vi "JSON Type Match.vi"(8 "error in (no error)":errorcluster, 9 "JSON Type":T1, 10 "JSON Value":string, 11 "Type":variant) -> (0 "error out":errorcluster, 1 "Types Match":bool, 2 "Variant Data String":string)   [LabVIEW 2011, in "LV JSON.lvlib"]
uses:
  LV JSON.lvlib
  <vilib>/Utility/VariantDataType/VariantType.lvlib
  <vilib>/picture/picture.llb/imagedata.ctl
  controls/JSON type.ctl
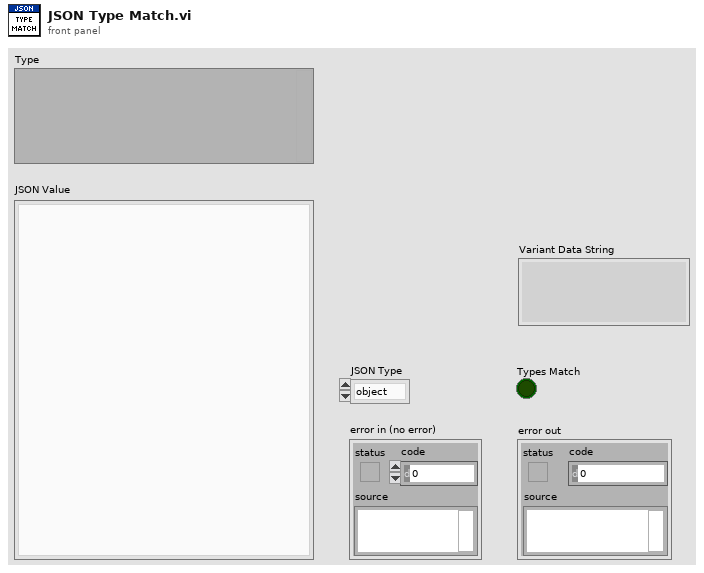
[diagram p1: front panel]
types:
  T1 = typedef "LV JSON.lvlib/JSON type.ctl" = enum16{"object", "array", "number", "string", "boolean", "null"}
  T2 = typedef "VariantType.lvlib/Type.ctl" = enum8{"Invalid Type", "Void", "I8", "I16", "I32", "I64", "U8", "U16", "U32", "U64", "Single Float", "Double Float", "Extended Float", "Single Complex", "Double Complex", "Extended Complex", "Enum U8", "Enum U16", "Enum U32", "Enum U64", "Single Float With Unit", "Double Float With Unit", "Extended Float With Unit", "Single Complex with Unit", "Double Complex with Unit", "Extended Complex with Unit", "Boolean", "String", "Path", "Picture", "Tag", "Array", "Cluster", "Variant", "LV Variant", "Waveform", "Timestamp", "Digital Waveform", "Digital Data", "ExpressData", "Refnum", "External Data", "VI", "Poly VI", "LabVIEW Class Instance", "Fixed Point"}
  T3 = typedef "imagedata.ctl" = cluster{"image type":i32, "image depth":i32, "image":u8[], "mask":u8[], "colors":u32[], "Rectangle":cluster{"left":i16, "top":i16, "right":i16, "bottom":i16}}
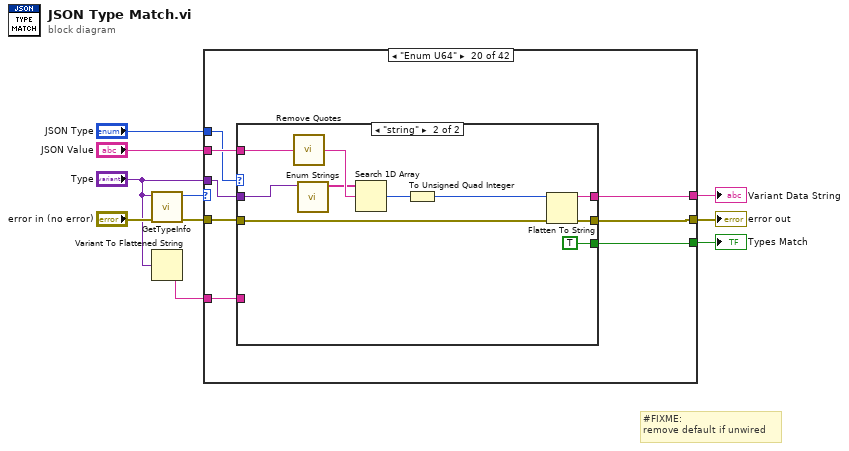
[diagram p0: block diagram]
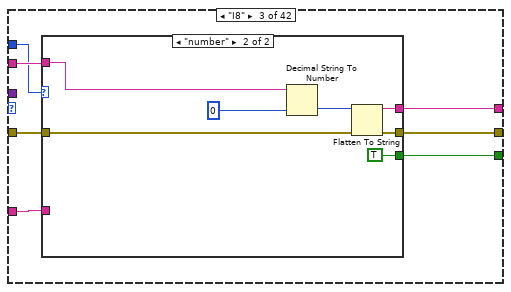
[diagram p4: hidden frame]
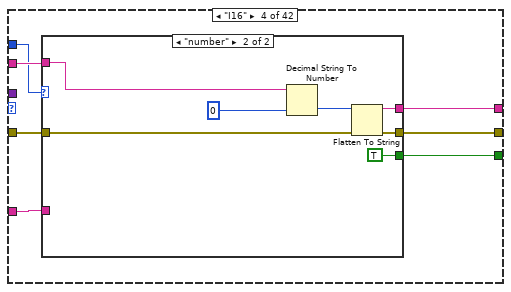
[diagram p6: hidden frame]
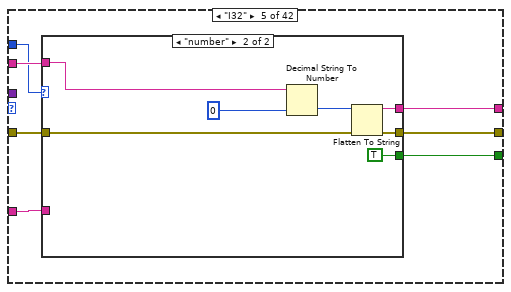
[diagram p8: hidden frame]
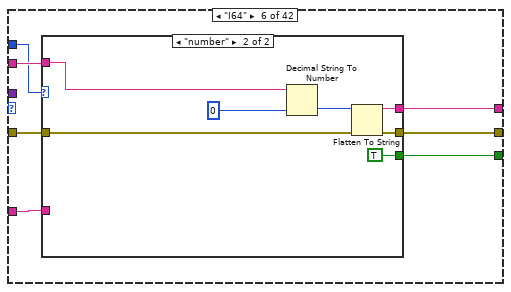
[diagram p10: hidden frame]
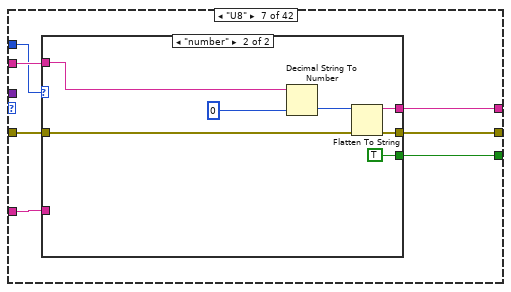
[diagram p12: hidden frame]
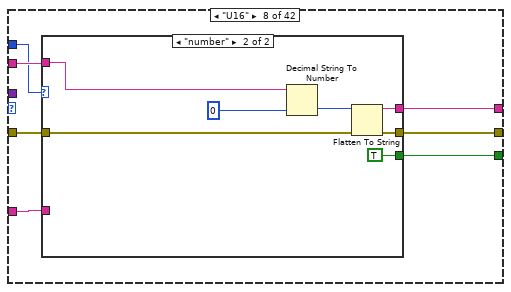
[diagram p14: hidden frame]
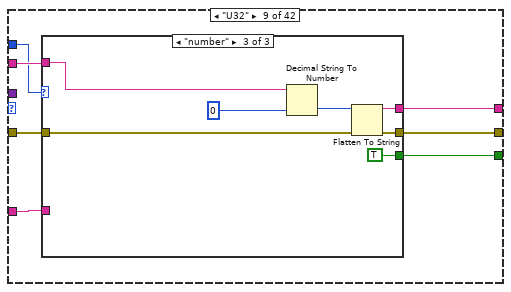
[diagram p16: hidden frame]
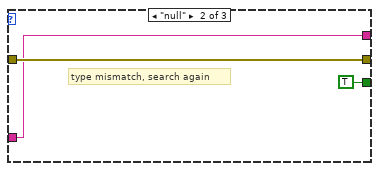
[diagram p18: hidden frame]
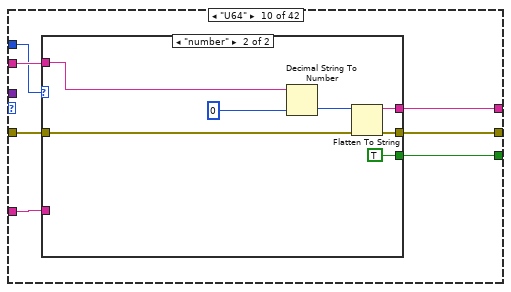
[diagram p19: hidden frame]
diagram:
  # "#FIXME:\nremove default if unwired"
  n1 = call <vilib>:"GetTypeInfo.vi"("error in (no error)"="error in (no error)", "Variant"="Type") -> ("error out"=w8:errorcluster, "Type Enum"=w7:T2)  [unwired: 5 in, 3 out]
  n2 = Variant To Flattened String(Variant="Type") -> (data string=w4:string)  [unwired: 1 out]
  n3 = case shown="\"Enum U64\"" w7 {
    tunnel: [_ _ w14 w30 w46 w62 w78 w94 w110 w129 w144 w164 w180 _ _ _ w191 w211 w231 w251 _ _ w272 w292 w296 w312 _ w326 w489 _ _ _ w510 _ _ _ w529 _ _ _ _ _] -> w1
    tunnel: w8 -> [_ _ w17 w33 w49 w65 w81 w97 w113 w132 w146 w163 w179 _ _ _ w196 w216 w236 w256 _ _ w274 w293 w298 w319 _ w328 w488 _ _ _ w509 _ _ _ w531 _ _ _ _ _]
    tunnel: [_ _ w13 w29 w45 w61 w77 w93 w109 w128 w142 w162 w178 _ _ _ w192 w212 w232 w252 _ _ w271 w291 w295 w313 _ w327 w487 _ _ _ w508 _ _ _ w531 _ _ _ _ _] -> w2
    tunnel: "Type" -> [_ _ _ _ _ _ _ _ _ _ _ _ _ _ _ _ w190 w210 w230 w250 _ _ _ _ _ _ _ w325 w482 _ _ _ _ _ _ _ _ _ _ _ _ _]
    tunnel: "JSON Value" -> [_ _ w16 w32 w48 w64 w80 w96 w112 w131 w148 w160 w176 _ _ _ w197 w217 w237 w257 _ _ w276 w289 w300 w320 _ w324 w485 _ _ _ w512 _ _ _ _ _ _ _ _ _]
    tunnel: "JSON Type" -> [_ _ w15 w31 w47 w63 w79 w95 w111 w130 w147 w161 w177 _ _ _ w194 w214 w234 w254 _ _ w275 _ w299 _ _ w323 w486 _ _ _ w511 _ _ _ _ _ _ _ _ _]
    tunnel: w4 -> [_ _ w11 w27 w43 w59 w75 w91 w107 w126 w145 w159 w175 _ _ _ w195 w215 w235 w255 _ _ w273 _ w297 _ _ w322 w484 _ _ _ w507 _ _ _ w529 _ _ _ _ _]
    tunnel: [_ _ w12 w28 w44 w60 w76 w92 w108 w127 w143 w158 w174 _ _ _ w193 w213 w233 w253 _ _ w270 TRUE w294 TRUE _ w321 w483 _ _ _ w513 _ _ _ TRUE _ _ _ _ _] -> w3
    frame "Invalid Type", Default {
    }
    frame "Void" {
    }
    frame "I8" {
      n4 = case shown="\"number\"" w15 {
        tunnel: [w18 w24] -> w14
        tunnel: w17 -> [w19 w23]
        tunnel: [w19 w22] -> w13
        tunnel: w16 -> [_ w21]
        tunnel: w11 -> [w18 _]
        tunnel: [_ TRUE] -> w12
        frame Default {
          # "type mismatch, search again"
        }
        frame "number" {
          n5 = Decimal String To Number(string=w21, default (0L)=i8 0 ("default (0 DBL)")) -> (number=w25:i8)  [unwired: 1 in, 1 out]
          n6 = Flatten To String(anything=w25, error in (no error)=w23) -> (data string=w24:string, error out=w22:errorcluster)  [unwired: 2 in, 1 out]
        }
      }
    }
    frame "I16" {
      n7 = case shown="\"number\"" w31 {
        tunnel: [w34 w40] -> w30
        tunnel: w33 -> [w35 w39]
        tunnel: [w35 w38] -> w29
        tunnel: w32 -> [_ w37]
        tunnel: w27 -> [w34 _]
        tunnel: [_ TRUE] -> w28
        frame Default {
          # "type mismatch, search again"
        }
        frame "number" {
          n8 = Decimal String To Number(string=w37, default (0L)=i16 0 ("default (0 DBL)")) -> (number=w41:i16)  [unwired: 1 in, 1 out]
          n9 = Flatten To String(anything=w41, error in (no error)=w39) -> (data string=w40:string, error out=w38:errorcluster)  [unwired: 2 in, 1 out]
        }
      }
    }
    frame "I32" {
      n10 = case shown="\"number\"" w47 {
        tunnel: [w50 w56] -> w46
        tunnel: w49 -> [w51 w55]
        tunnel: [w51 w54] -> w45
        tunnel: w48 -> [_ w53]
        tunnel: w43 -> [w50 _]
        tunnel: [_ TRUE] -> w44
        frame Default {
          # "type mismatch, search again"
        }
        frame "number" {
          n11 = Decimal String To Number(string=w53, default (0L)=0 ("default (0 DBL)")) -> (number=w57:i32)  [unwired: 1 in, 1 out]
          n12 = Flatten To String(anything=w57, error in (no error)=w55) -> (data string=w56:string, error out=w54:errorcluster)  [unwired: 2 in, 1 out]
        }
      }
    }
    frame "I64" {
      n13 = case shown="\"number\"" w63 {
        tunnel: [w66 w72] -> w62
        tunnel: w65 -> [w67 w71]
        tunnel: [w67 w70] -> w61
        tunnel: w64 -> [_ w69]
        tunnel: w59 -> [w66 _]
        tunnel: [_ TRUE] -> w60
        frame Default {
          # "type mismatch, search again"
        }
        frame "number" {
          n14 = Decimal String To Number(string=w69, default (0L)=i64 0 ("default (0 DBL)")) -> (number=w73:i64)  [unwired: 1 in, 1 out]
          n15 = Flatten To String(anything=w73, error in (no error)=w71) -> (data string=w72:string, error out=w70:errorcluster)  [unwired: 2 in, 1 out]
        }
      }
    }
    frame "U8" {
      n16 = case shown="\"number\"" w79 {
        tunnel: [w82 w88] -> w78
        tunnel: w81 -> [w83 w87]
        tunnel: [w83 w86] -> w77
        tunnel: w80 -> [_ w85]
        tunnel: w75 -> [w82 _]
        tunnel: [_ TRUE] -> w76
        frame Default {
          # "type mismatch, search again"
        }
        frame "number" {
          n17 = Decimal String To Number(string=w85, default (0L)=u8 0 ("default (0 DBL)")) -> (number=w89:u8)  [unwired: 1 in, 1 out]
          n18 = Flatten To String(anything=w89, error in (no error)=w87) -> (data string=w88:string, error out=w86:errorcluster)  [unwired: 2 in, 1 out]
        }
      }
    }
    frame "U16" {
      n19 = case shown="\"number\"" w95 {
        tunnel: [w98 w104] -> w94
        tunnel: w97 -> [w99 w103]
        tunnel: [w99 w102] -> w93
        tunnel: w96 -> [_ w101]
        tunnel: w91 -> [w98 _]
        tunnel: [_ TRUE] -> w92
        frame Default {
          # "type mismatch, search again"
        }
        frame "number" {
          n20 = Decimal String To Number(string=w101, default (0L)=u16 0 ("default (0 DBL)")) -> (number=w105:u16)  [unwired: 1 in, 1 out]
          n21 = Flatten To String(anything=w105, error in (no error)=w103) -> (data string=w104:string, error out=w102:errorcluster)  [unwired: 2 in, 1 out]
        }
      }
    }
    frame "U32" {
      n22 = case shown="\"number\"" w111 {
        tunnel: [w114 w117 w123] -> w110
        tunnel: w113 -> [w115 w118 w122]
        tunnel: [w115 w118 w121] -> w109
        tunnel: w112 -> [_ _ w120]
        tunnel: w107 -> [w114 w117 _]
        tunnel: [_ TRUE TRUE] -> w108
        frame Default {
          # "type mismatch, search again"
        }
        frame "null" {
          # "type mismatch, search again"
        }
        frame "number" {
          n23 = Decimal String To Number(string=w120, default (0L)=u32 0 ("default (0 DBL)")) -> (number=w124:u32)  [unwired: 1 in, 1 out]
          n24 = Flatten To String(anything=w124, error in (no error)=w122) -> (data string=w123:string, error out=w121:errorcluster)  [unwired: 2 in, 1 out]
        }
      }
    }
    frame "U64" {
      n25 = case shown="\"number\"" w130 {
        tunnel: [w133 w139] -> w129
        tunnel: w132 -> [w134 w138]
        tunnel: [w134 w137] -> w128
        tunnel: w131 -> [_ w136]
        tunnel: w126 -> [w133 _]
        tunnel: [_ TRUE] -> w127
        frame Default {
          # "type mismatch, search again"
        }
        frame "number" {
          n26 = Decimal String To Number(string=w136, default (0L)=u64 0 ("default (0 DBL)")) -> (number=w140:u64)  [unwired: 1 in, 1 out]
          n27 = Flatten To String(anything=w140, error in (no error)=w138) -> (data string=w139:string, error out=w137:errorcluster)  [unwired: 2 in, 1 out]
        }
      }
    }
    frame "Single Float", "Single Float With Unit" {
      n28 = case shown="\"number\"" w147 {
        tunnel: [w149 w155] -> w144
        tunnel: w146 -> [w150 w154]
        tunnel: [w150 w153] -> w142
        tunnel: w148 -> [_ w152]
        tunnel: w145 -> [w149 _]
        tunnel: [_ TRUE] -> w143
        frame Default {
          # "type mismatch, search again"
        }
        frame "number" {
          n29 = Fract/Exp String To Number(string=w152, default (0 dbl)=sgl 0.0 ("default (0 DBL)")) -> (number=w156:sgl)  [unwired: 2 in, 1 out]
          n30 = Flatten To String(anything=w156, error in (no error)=w154) -> (data string=w155:string, error out=w153:errorcluster)  [unwired: 2 in, 1 out]
        }
      }
    }
    frame "Double Float", "Double Float With Unit" {
      n31 = case shown="\"number\"" w161 {
        tunnel: [w165 w171] -> w164
        tunnel: w163 -> [w166 w170]
        tunnel: [w166 w169] -> w162
        tunnel: w160 -> [_ w168]
        tunnel: w159 -> [w165 _]
        tunnel: [_ TRUE] -> w158
        frame Default {
          # "type mismatch, search again"
        }
        frame "number" {
          n32 = Fract/Exp String To Number(string=w168, default (0 dbl)=0.0 ("default (0 DBL)")) -> (number=w172:dbl)  [unwired: 2 in, 1 out]
          n33 = Flatten To String(anything=w172, error in (no error)=w170) -> (data string=w171:string, error out=w169:errorcluster)  [unwired: 2 in, 1 out]
        }
      }
    }
    frame "Extended Float", "Extended Float With Unit" {
      n34 = case shown="\"number\"" w177 {
        tunnel: [w181 w187] -> w180
        tunnel: w179 -> [w182 w186]
        tunnel: [w182 w185] -> w178
        tunnel: w176 -> [_ w184]
        tunnel: w175 -> [w181 _]
        tunnel: [_ TRUE] -> w174
        frame Default {
          # "type mismatch, search again"
        }
        frame "number" {
          n35 = Fract/Exp String To Number(string=w184, default (0 dbl)=ext 0.0 ("default (0 DBL)")) -> (number=w188:ext)  [unwired: 2 in, 1 out]
          n36 = Flatten To String(anything=w188, error in (no error)=w186) -> (data string=w187:string, error out=w185:errorcluster)  [unwired: 2 in, 1 out]
        }
      }
    }
    frame "Single Complex" {
    }
    frame "Double Complex" {
    }
    frame "Extended Complex" {
    }
    frame "Enum U8" {
      n37 = case shown="\"string\"" w194 {
        tunnel: [w198 w207] -> w191
        tunnel: w196 -> [w199 w200]
        tunnel: [w199 w208] -> w192
        tunnel: w197 -> [_ w204]
        tunnel: w195 -> [w198 _]
        tunnel: [_ TRUE] -> w193
        tunnel: w190 -> [_ w202]
        frame Default {
          # "type mismatch, search again"
        }
        frame "string" {
          n38 = call "Remove Quotes.vi"("String"=w204) -> ("String without Quotes"=w203:string)
          n39 = call "Enum Strings.vi"("Enum"=w202) -> ("Strings"=w201:string[])  [unwired: 8 in, 2 out]
          n40 = Search 1D Array(1D array=w201, element=w203) -> (index of element=w206:i32)  [unwired: 1 in]
          n41 = To Unsigned Byte Integer(number=w206) -> (unsigned 8bit integer=w205:u8)
          n42 = Flatten To String(anything=w205, error in (no error)=w200) -> (data string=w207:string, error out=w208:errorcluster)  [unwired: 2 in, 1 out]
        }
      }
    }
    frame "Enum U16" {
      n43 = case shown="\"string\"" w214 {
        tunnel: [w218 w227] -> w211
        tunnel: w216 -> [w219 w220]
        tunnel: [w219 w228] -> w212
        tunnel: w217 -> [_ w224]
        tunnel: w215 -> [w218 _]
        tunnel: [_ TRUE] -> w213
        tunnel: w210 -> [_ w222]
        frame Default {
          # "type mismatch, search again"
        }
        frame "string" {
          n44 = call "Remove Quotes.vi"("String"=w224) -> ("String without Quotes"=w223:string)
          n45 = call "Enum Strings.vi"("Enum"=w222) -> ("Strings"=w221:string[])  [unwired: 8 in, 2 out]
          n46 = Search 1D Array(1D array=w221, element=w223) -> (index of element=w226:i32)  [unwired: 1 in]
          n47 = To Unsigned Word Integer(number=w226) -> (unsigned 16bit integer=w225:u16)
          n48 = Flatten To String(anything=w225, error in (no error)=w220) -> (data string=w227:string, error out=w228:errorcluster)  [unwired: 2 in, 1 out]
        }
      }
    }
    frame "Enum U32" {
      n49 = case shown="\"string\"" w234 {
        tunnel: [w238 w247] -> w231
        tunnel: w236 -> [w239 w240]
        tunnel: [w239 w248] -> w232
        tunnel: w237 -> [_ w244]
        tunnel: w235 -> [w238 _]
        tunnel: [_ TRUE] -> w233
        tunnel: w230 -> [_ w241]
        frame Default {
          # "type mismatch, search again"
        }
        frame "string" {
          n50 = call "Remove Quotes.vi"("String"=w244) -> ("String without Quotes"=w243:string)
          n51 = call "Enum Strings.vi"("Enum"=w241) -> ("Strings"=w242:string[])  [unwired: 8 in, 2 out]
          n52 = Search 1D Array(1D array=w242, element=w243) -> (index of element=w246:i32)  [unwired: 1 in]
          n53 = To Unsigned Long Integer(number=w246) -> (unsigned 32bit integer=w245:u32)
          n54 = Flatten To String(anything=w245, error in (no error)=w240) -> (data string=w247:string, error out=w248:errorcluster)  [unwired: 2 in, 1 out]
        }
      }
    }
    frame "Enum U64" {
      n55 = case shown="\"string\"" w254 {
        tunnel: [w258 w267] -> w251
        tunnel: w256 -> [w259 w261]
        tunnel: [w259 w268] -> w252
        tunnel: w257 -> [_ w264]
        tunnel: w255 -> [w258 _]
        tunnel: [_ TRUE] -> w253
        tunnel: w250 -> [_ w260]
        frame Default {
          # "type mismatch, search again"
        }
        frame "string" {
          n56 = call "Remove Quotes.vi"("String"=w264) -> ("String without Quotes"=w263:string)
          n57 = call "Enum Strings.vi"("Enum"=w260) -> ("Strings"=w262:string[])  [unwired: 8 in, 2 out]
          n58 = Search 1D Array(1D array=w262, element=w263) -> (index of element=w266:i32)  [unwired: 1 in]
          n59 = To Unsigned Quad Integer(1:w266) -> (0:w265:u64)
          n60 = Flatten To String(anything=w265, error in (no error)=w261) -> (data string=w267:string, error out=w268:errorcluster)  [unwired: 2 in, 1 out]
        }
      }
    }
    frame "Single Complex with Unit" {
    }
    frame "Extended Complex with Unit" {
    }
    frame "Boolean" {
      n61 = case shown="\"boolean\"" w275 {
        tunnel: [w277 w282] -> w272
        tunnel: w274 -> [w278 w280]
        tunnel: [w278 w283] -> w271
        tunnel: w276 -> [_ w285]
        tunnel: w273 -> [w277 _]
        tunnel: [_ TRUE] -> w270
        frame Default {
          # "type mismatch, search again"
        }
        frame "boolean" {
          n62 = To Lower Case(string=w285) -> (all lower case string=w279:string)
          n63 = Equal?(x=w279, y="true") -> (x = y?=w281:bool)
          n64 = Flatten To String(anything=w281, error in (no error)=w280) -> (data string=w282:string, error out=w283:errorcluster)  [unwired: 2 in, 1 out]
        }
      }
    }
    frame "String" {
      n65 = call "Remove Quotes.vi"("String"=w289) -> ("String without Quotes"=w288:string)
      n66 = call "JSON Unescape.vi"("Escaped JSON String"=w288) -> ("JSON String"=w287:string)
      n67 = Flatten To String(anything=w287, error in (no error)=w293) -> (data string=w292:string, error out=w291:errorcluster)  [unwired: 2 in, 1 out]
    }
    frame "Path" {
      n68 = case shown="\"string\"" w299 {
        tunnel: [w301 w310] -> w296
        tunnel: w298 -> [w302 w309]
        tunnel: [w302 w308] -> w295
        tunnel: w300 -> [_ w305]
        tunnel: w297 -> [w301 _]
        tunnel: [_ TRUE] -> w294
        frame Default {
          # "type mismatch, search again"
        }
        frame "string" {
          n69 = call "Remove Quotes.vi"("String"=w305) -> ("String without Quotes"=w304:string)
          n70 = call "JSON Unescape.vi"("Escaped JSON String"=w304) -> ("JSON String"=w303:string)
          n71 = String To Path(string=w303) -> (path=w306:path)
          n72 = Flatten To String(anything=w306, error in (no error)=w309) -> (data string=w310:string, error out=w308:errorcluster)  [unwired: 2 in, 1 out]
        }
      }
    }
    frame "Picture" {
      w317 = T3 {"image type"=0, "image depth"=0, "image"=[], "mask"=[], "colors"=[], "Rectangle"={"left"=0, "top"=0, "right"=0, "bottom"=0}} ("image data")
      n73 = call "JSON to Anything.vi"("error in (no error)"=w319, "JSON Object"=w320, "Type"=w317) -> ("error out"=w316:errorcluster, "Variant"=w318:variant)  [unwired: 5 in, 2 out]
      n74 = Variant To Data(error in=w316, type=w317, Variant=w318) -> (data=w314:T3, error out=w315:errorcluster)
      n75 = Flatten To String(anything=w314, error in (no error)=w315) -> (data string=w312:string, error out=w313:errorcluster)  [unwired: 2 in, 1 out]
    }
    frame "Tag" {
    }
    frame "Array" {
      n76 = case shown="\"array\"" w323 {
        tunnel: w328 -> [w330 w339]
        tunnel: [w330 w334] -> w327
        tunnel: [w329 w333] -> w326
        tunnel: w325 -> [_ w337]
        tunnel: w324 -> [_ w331]
        tunnel: w322 -> [w329 _]
        tunnel: [_ TRUE] -> w321
        frame Default {
        }
        frame "array" {
          n77 = call "JSON Parse Array.vi"("error in (no error)"=w339, "JSON Array Value"=w331, "Type"=w337) -> ("error out"=w338:errorcluster, "variant"=w335:variant, "Type Enum"=w332:T2)  [unwired: 5 in, 1 out]
          n78 = case shown="\"Cluster\"" w332 {
            tunnel: w338 -> [w340 w347 w354 w361 w368 w375 w382 w389 w396 w403 w410 w417 w424 w431 w438 w445 w452 w459 w464]
            tunnel: w335 -> [_ w346 w353 w360 w367 w374 w381 w388 w395 w402 w409 w416 w423 w430 w437 w444 w451 w458 w463]
            tunnel: [w340 w343 w350 w357 w364 w371 w378 w385 w392 w399 w406 w413 w420 w427 w434 w442 w449 w456 w460] -> w334
            tunnel: [_ w342 w349 w356 w363 w370 w377 w384 w391 w398 w405 w412 w419 w426 w433 w441 w448 w455 w461] -> w333
            tunnel: w331 -> [_ _ _ _ _ _ _ _ _ _ _ _ _ _ _ _ _ _ w462]
            frame "Invalid Type", Default {
            }
            frame "Double Float", "Double Float With Unit" {
              n79 = Variant To Data(error in=w347, type=dbl[] [], Variant=w346) -> (data=w341:dbl[], error out=w344:errorcluster)
              n80 = Flatten To String(anything=w341, error in (no error)=w344) -> (data string=w342:string, error out=w343:errorcluster)  [unwired: 2 in, 1 out]
            }
            frame "Single Float", "Single Float With Unit" {
              n81 = Variant To Data(error in=w354, type=sgl[] [], Variant=w353) -> (data=w348:sgl[], error out=w351:errorcluster)
              n82 = Flatten To String(anything=w348, error in (no error)=w351) -> (data string=w349:string, error out=w350:errorcluster)  [unwired: 2 in, 1 out]
            }
            frame "Extended Float", "Extended Float With Unit" {
              n83 = Variant To Data(error in=w361, type=ext[] [], Variant=w360) -> (data=w355:ext[], error out=w358:errorcluster)
              n84 = Flatten To String(anything=w355, error in (no error)=w358) -> (data string=w356:string, error out=w357:errorcluster)  [unwired: 2 in, 1 out]
            }
            frame "Single Complex" {
              n85 = Variant To Data(error in=w368, type=csg[] [], Variant=w367) -> (data=w362:csg[], error out=w365:errorcluster)
              n86 = Flatten To String(anything=w362, error in (no error)=w365) -> (data string=w363:string, error out=w364:errorcluster)  [unwired: 2 in, 1 out]
            }
            frame "Double Complex" {
              n87 = Variant To Data(error in=w375, type=cdb[] [], Variant=w374) -> (data=w369:cdb[], error out=w372:errorcluster)
              n88 = Flatten To String(anything=w369, error in (no error)=w372) -> (data string=w370:string, error out=w371:errorcluster)  [unwired: 2 in, 1 out]
            }
            frame "Extended Complex" {
              n89 = Variant To Data(error in=w382, type=cxt[] [], Variant=w381) -> (data=w376:cxt[], error out=w379:errorcluster)
              n90 = Flatten To String(anything=w376, error in (no error)=w379) -> (data string=w377:string, error out=w378:errorcluster)  [unwired: 2 in, 1 out]
            }
            frame "I8" {
              n91 = Variant To Data(error in=w389, type=i8[] [], Variant=w388) -> (data=w383:i8[], error out=w386:errorcluster)
              n92 = Flatten To String(anything=w383, error in (no error)=w386) -> (data string=w384:string, error out=w385:errorcluster)  [unwired: 2 in, 1 out]
            }
            frame "I16" {
              n93 = Variant To Data(error in=w396, type=i16[] [], Variant=w395) -> (data=w390:i16[], error out=w393:errorcluster)
              n94 = Flatten To String(anything=w390, error in (no error)=w393) -> (data string=w391:string, error out=w392:errorcluster)  [unwired: 2 in, 1 out]
            }
            frame "I32" {
              n95 = Variant To Data(error in=w403, type=i32[] [], Variant=w402) -> (data=w397:i32[], error out=w400:errorcluster)
              n96 = Flatten To String(anything=w397, error in (no error)=w400) -> (data string=w398:string, error out=w399:errorcluster)  [unwired: 2 in, 1 out]
            }
            frame "I64" {
              n97 = Variant To Data(error in=w410, type=i64[] [], Variant=w409) -> (data=w404:i64[], error out=w407:errorcluster)
              n98 = Flatten To String(anything=w404, error in (no error)=w407) -> (data string=w405:string, error out=w406:errorcluster)  [unwired: 2 in, 1 out]
            }
            frame "U8" {
              n99 = Variant To Data(error in=w417, type=u8[] [], Variant=w416) -> (data=w411:u8[], error out=w414:errorcluster)
              n100 = Flatten To String(anything=w411, error in (no error)=w414) -> (data string=w412:string, error out=w413:errorcluster)  [unwired: 2 in, 1 out]
            }
            frame "U16" {
              n101 = Variant To Data(error in=w424, type=u16[] [], Variant=w423) -> (data=w418:u16[], error out=w421:errorcluster)
              n102 = Flatten To String(anything=w418, error in (no error)=w421) -> (data string=w419:string, error out=w420:errorcluster)  [unwired: 2 in, 1 out]
            }
            frame "U32" {
              n103 = Variant To Data(error in=w431, type=u32[] [], Variant=w430) -> (data=w425:u32[], error out=w428:errorcluster)
              n104 = Flatten To String(anything=w425, error in (no error)=w428) -> (data string=w426:string, error out=w427:errorcluster)  [unwired: 2 in, 1 out]
            }
            frame "U64" {
              n105 = Variant To Data(error in=w438, type=u64[] [], Variant=w437) -> (data=w432:u64[], error out=w435:errorcluster)
              n106 = Flatten To String(anything=w432, error in (no error)=w435) -> (data string=w433:string, error out=w434:errorcluster)  [unwired: 2 in, 1 out]
            }
            frame "Path" {
              n107 = Variant To Data(error in=w445, type=path[] [], Variant=w444) -> (data=w440:path[], error out=w443:errorcluster)
              n108 = Flatten To String(anything=w440, error in (no error)=w443) -> (data string=w441:string, error out=w442:errorcluster)  [unwired: 2 in, 1 out]
            }
            frame "Boolean" {
              n109 = Variant To Data(error in=w452, type=bool[] [], Variant=w451) -> (data=w447:bool[], error out=w450:errorcluster)
              n110 = Flatten To String(anything=w447, error in (no error)=w450) -> (data string=w448:string, error out=w449:errorcluster)  [unwired: 2 in, 1 out]
            }
            frame "String" {
              n111 = Variant To Data(error in=w459, type=string[] [], Variant=w458) -> (data=w454:string[], error out=w457:errorcluster)
              n112 = Flatten To String(anything=w454, error in (no error)=w457) -> (data string=w455:string, error out=w456:errorcluster)  [unwired: 2 in, 1 out]
            }
            frame "Cluster" {
              n113 = disable-structure shown="Enabled" {
                disable-tunnel: w464 -> [w471 w480]
                disable-tunnel: w463 -> [w470 w481]
                disable-tunnel: w462 -> [w469 _]
                disable-tunnel: [w466 w479] -> w461
                disable-tunnel: [w465 w480] -> w460
                frame Disabled {
                  n114 = call "Cluster Elements.vi"("error in (no error)"=w471, "Cluster Variant"=w470) -> ("error out"=w472:errorcluster, "Cluster Elements"=w473:variant[])  [unwired: 8 in]
                  n115 = for {
                    tunnel: w472 -> [w478]
                    tunnel: w473 -> [w475] mode=indexing
                    tunnel: w469 -> [w474]
                    tunnel: [w477] -> w468 mode=indexing
                    tunnel: [w476] -> w467 mode=indexing
                    n116 = call "JSON to Anything.vi"("error in (no error)"=w478, "JSON Object"=w474, "Type"=w475) -> ("error out"=w477:errorcluster, "Variant Data String"=w476:string)  [unwired: 5 in, 2 out]
                  }
                  n117 = Concatenate Strings(w467) -> (w466:string)
                  n118 = Merge Errors(w468) -> (w465:errorcluster)
                }
                frame Enabled {
                  n119 = Variant To Flattened String(Variant=w481) -> (data string=w479:string)  [unwired: 1 out]
                }
              }
            }
          }
        }
      }
    }
    frame "Cluster" {
      n120 = case shown="\"object\"" w486 {
        tunnel: [w490 w494] -> w489
        tunnel: w488 -> [w491 w500]
        tunnel: [w491 w492] -> w487
        tunnel: w485 -> [_ w496]
        tunnel: w484 -> [w490 _]
        tunnel: [_ TRUE] -> w483
        tunnel: w482 -> [_ w499]
        frame Default {
        }
        frame "object" {
          n121 = call "Cluster Elements.vi"("error in (no error)"=w500, "Cluster Variant"=w499) -> ("error out"=w498:errorcluster, "Cluster Elements"=w497:variant[])  [unwired: 8 in]
          n122 = for {
            tunnel: w498 -> [w506]
            tunnel: w497 -> [w503] mode=indexing
            tunnel: w496 -> [w502]
            tunnel: [w505] -> w493 mode=indexing
            tunnel: [w504] -> w495 mode=indexing
            n123 = call "JSON to Anything.vi"("error in (no error)"=w506, "JSON Object"=w502, "Type"=w503) -> ("error out"=w505:errorcluster, "Variant Data String"=w504:string)  [unwired: 5 in, 2 out]
          }
          n124 = Concatenate Strings(w495) -> (w494:string)
          n125 = Merge Errors(w493) -> (w492:errorcluster)
        }
      }
    }
    frame "Variant" {
    }
    frame "LV Variant" {
    }
    frame "Waveform" {
    }
    frame "Timestamp" {
      n126 = case shown="\"string\"" w511 {
        tunnel: [w514 w516 w528] -> w510
        tunnel: w509 -> [w515 w518 w527]
        tunnel: [w515 w518 w526] -> w508
        tunnel: w512 -> [_ _ w524]
        tunnel: [_ TRUE TRUE] -> w513
        tunnel: w507 -> [w514 w516 _]
        frame Default {
          # "type mismatch, search again"
        }
        frame "null" {
          # "type mismatch, search again"
        }
        frame "string" {
          n127 = call "Remove Quotes.vi"("String"=w524) -> ("String without Quotes"=w520:string)
          n128 = call "JSON Unescape.vi"("Escaped JSON String"=w520) -> ("JSON String"=w519:string)
          n129 = Scan From String(format string="%<%02m/%02d/%Y %H:%M:%S%03u>T", input string=w519, default 1=timestamp(0 s since 1904-01-01) ("time stamp")) -> (output 1=w521:timestamp)  [unwired: 2 in, 3 out]
          n130 = Flatten To String(anything=w521, error in (no error)=w527) -> (data string=w528:string, error out=w526:errorcluster)  [unwired: 2 in, 1 out]
        }
      }
    }
    frame "Digital Waveform" {
    }
    frame "Digital Data" {
    }
    frame "ExpressData" {
    }
    frame "Refnum" {
    }
    frame "External Data" {
    }
    frame "VI" {
    }
    frame "Poly VI" {
    }
    frame "LabVIEW Class Instance" {
    }
    frame "Fixed Point" {
    }
  }
  "Types Match" <- w3
  "error out" <- w2
  "Variant Data String" <- w1
